vi "dfd_Utility I32 x I16 (MSBs).vi"(1 "y[I16]":i16, 2 "x[I32]":i32) -> (0 "x*y[I32 MSB]":i32)   [LabVIEW 2017, in "NI_DigFilterLicensed.lvlib"]
uses:
  <vilib>/addons/Digital Filter Design/NI_DigFilterLicensed.lvlib
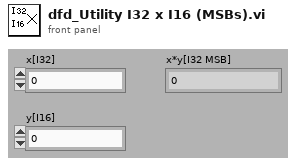
[diagram p1: front panel]
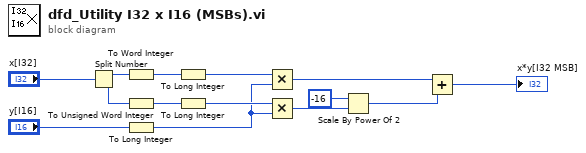
[diagram p0: block diagram]
diagram:
  n1 = Split Number(x="x[I32]") -> (hi(x)=w14:u16, lo(x)=w12:u16)
  n2 = To Word Integer(number=w14) -> (16bit integer=w10:i16)
  n3 = To Unsigned Word Integer(number=w12) -> (unsigned 16bit integer=w9:u16)
  n4 = To Long Integer(number="y[I16]") -> (32bit integer=w6:i32)
  n5 = To Long Integer(number=w10) -> (32bit integer=w8:i32)
  n6 = To Long Integer(number=w9) -> (32bit integer=w7:i32)
  n7 = Multiply(x=w8, y=w6) -> (x*y=w5:i32)
  n8 = Multiply(x=w7, y=w6) -> (x*y=w3:i32)
  n9 = Scale By Power Of 2(n=-16, x=w3) -> (x*2^n=w1:i32)
  n10 = Add(x=w5, y=w1) -> (x+y=→"x*y[I32 MSB]":i32)
